vi "PrefDialog.vi"(8 "error in (no error)":errorcluster, 11 "MyPluginsBase in":refnum<class "MyPluginsBase.lvclass">) -> (0 "error out":errorcluster, 3 "MyPluginsBase out":refnum<class "MyPluginsBase.lvclass">)   [LabVIEW 2014, in "MyPlugins.lvlib" / "MyPluginsBase.lvclass"]
uses:
  MyPluginsBase.lvclass
panel:
  in  "btnCancel":bool
  # "This Plugin has no configurable preferences"
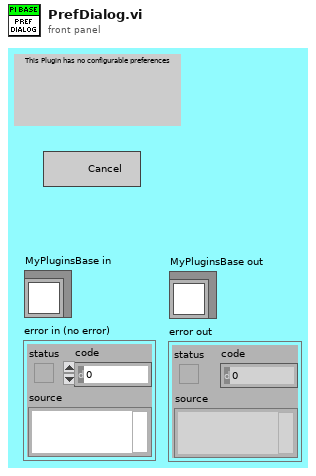
[diagram p1: front panel]
types:
  T1 = enum32{"Invalid", "Default", "Floating", "Floating/Auto-Hide", "Modal"}
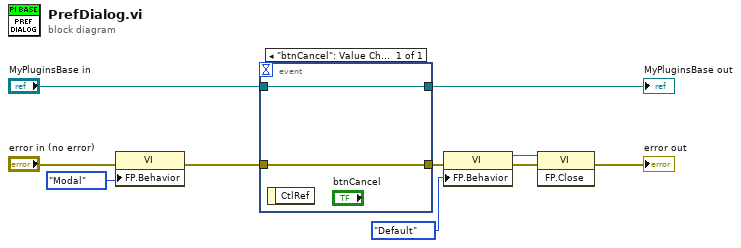
[diagram p0: block diagram]
diagram:
  n1 = property class="VI"(error in="error in (no error)", "FP.Behavior"=T1."Modal" ("Front Panel Window:Behavior")) -> (error out=w7:errorcluster)  [unwired: 1 in, 1 out]
  n2 = event shown="[0] \"btnCancel\": Value Change" {
    selector: _ -> [_]
    dyn-events: _ -> [_]
    timeout: _ -> [_]
    tunnel: "MyPluginsBase in" -> [w12]
    tunnel: [w12] -> w9
    tunnel: [w11] -> w5
    tunnel: w7 -> [w11]
    event "btnCancel": Value Change {
      n3 = event-data() -> ()  [unwired: 1 in, 1 out]
    }
  }
  "MyPluginsBase out" <- w9
  n4 = property class="VI"(error in=w5, "FP.Behavior"=T1."Default" ("Front Panel Window:Behavior")) -> (reference out=w1:refnum<vi>, error out=w4:errorcluster)  [unwired: 1 in]
  n5 = invoke class="VI" method="FP.Close"(reference=w1, error in=w4) -> (error out=→"error out":errorcluster)  [unwired: 1 in, 2 out]
